vi "ControlXY.vi"(6 "Y":string, 7 "X":string, 9 "Move?":bool, 10 "Reset":bool) -> ()   [LabVIEW 2014]
panel:
  in  "stop":bool
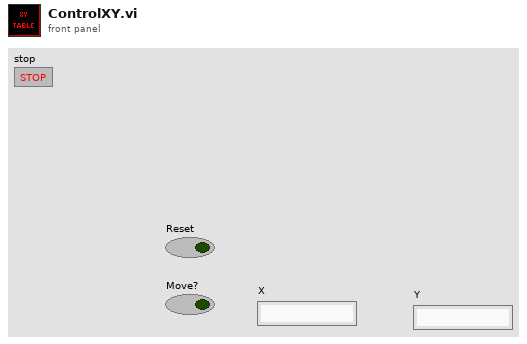
[diagram p1: front panel]
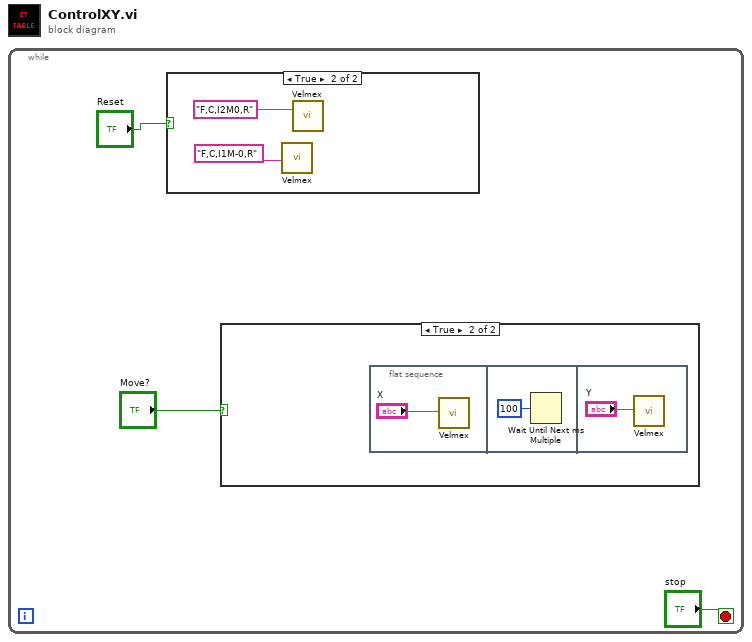
[diagram p0: block diagram]
diagram:
  n1 = while {
    stop <- "stop" stop-if-true
    n2 = case shown="True" "Reset" {
      frame False {
      }
      frame True {
        n3 = call "Velmex.Vi"("Command String"="F,C,I1M-0,R" ("X 2")) -> ()  [unwired: 6 in]
        n4 = call "Velmex.Vi"("Command String"="F,C,I2M0,R" ("Y 2")) -> ()  [unwired: 6 in]
      }
    }
    n5 = case shown="True" "Move?" {
      frame False {
      }
      frame True {
        n6 = flat-sequence {
          frame #0 {
            n7 = call "Velmex.Vi"("Command String"="X") -> ()  [unwired: 6 in]
          }
          frame #1 {
            n8 = Wait Until Next ms Multiple(millisecond multiple=u32 100) -> ()  [unwired: 1 out]
          }
          frame #2 {
            n9 = call "Velmex.Vi"("Command String"="Y") -> ()  [unwired: 6 in]
          }
        }
      }
    }
  }
